vi "User Update.vi"(8 "error in (no error)":errorcluster, 10 "User Record":T2, 11 "Connection Refnum":T1) -> (0 "error out":errorcluster, 3 "dup Connection Refnum":T1)   [LabVIEW 2011]
uses:
  User Record.ctl
  SI.LIB/ODBC/SQL Controls/Connection Refnum.ctl
panel:
  out "resulting string":string
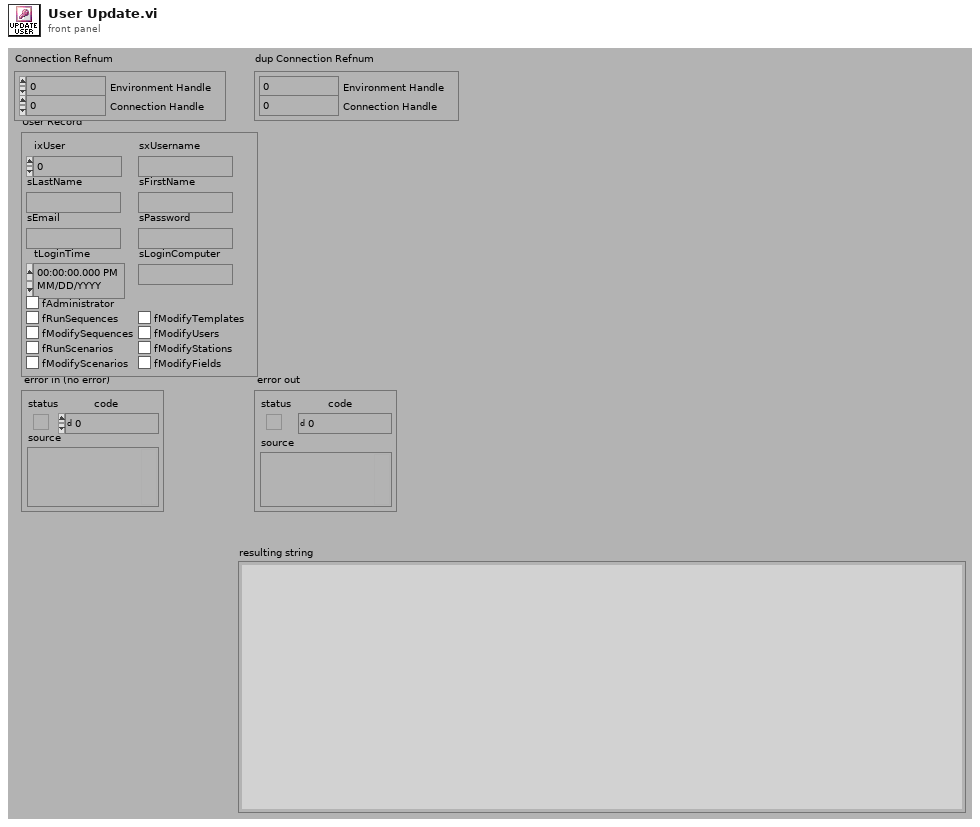
[diagram p1: front panel]
types:
  T1 = typedef "Connection Refnum.ctl" = cluster{"Environment Handle":i32, "Connection Handle":i32}
  T2 = typedef "User Record.ctl" = cluster{"ixUser":i32, "sxUsername":string, "sLastName":string, "sFirstName":string, "sEmail":string, "sPassword":string, "tLoginTime":timestamp, "sLoginComputer":string, "fAdministrator":bool, "fRunSequences":bool, "fModifySequences":bool, "fRunScenarios":bool, "fModifyScenarios":bool, "fModifyTemplates":bool, "fModifyUsers":bool, "fModifyStations":bool, "fModifyFields":bool}
  T3 = typedef "Statement Refnum.ctl" = cluster{"Statement Handle":i32, "Parameter Number":u16}
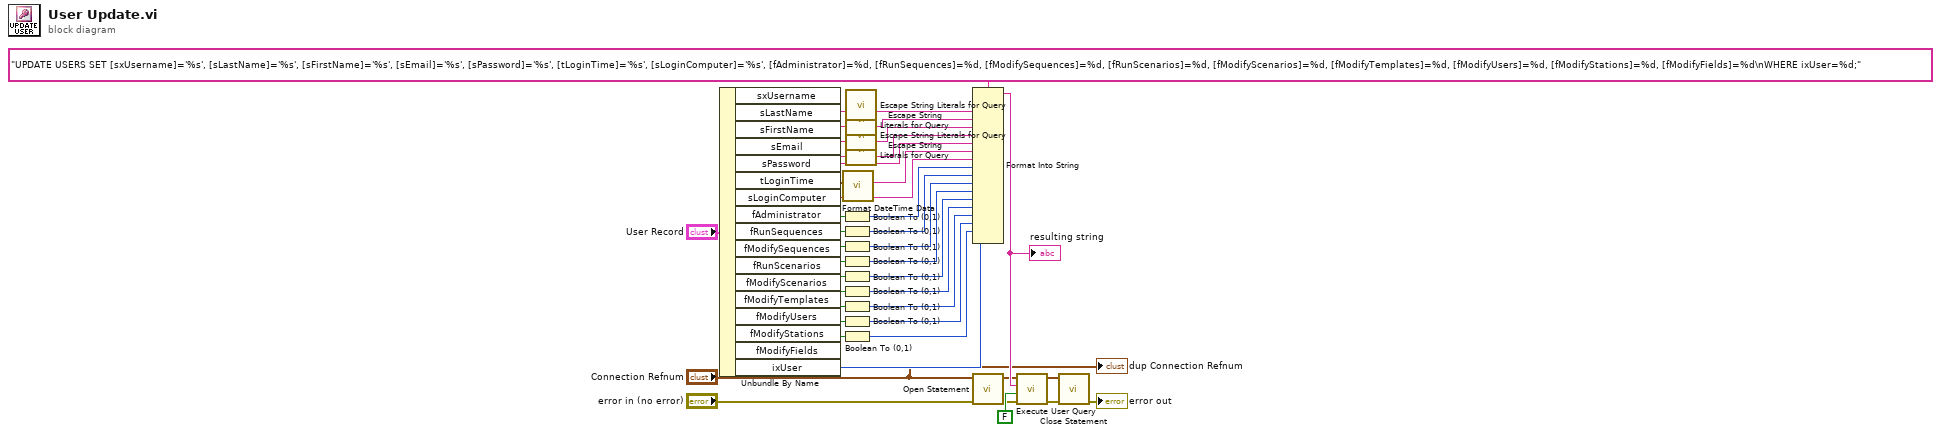
[diagram p0: block diagram]
diagram:
  n1 = Unbundle By Name("User Record") -> ("sxUsername"=w32:string, "sLastName"=w28:string, "sFirstName"=w29:string, "sEmail"=w30:string, "sPassword"=w23:string, "tLoginTime"=w27:timestamp, "sLoginComputer"=w34:string, "fAdministrator"=w20:bool, "fRunSequences"=w19:bool, "fModifySequences"=w18:bool, "fRunScenarios"=w14:bool, "fModifyScenarios"=w13:bool, "fModifyTemplates"=w12:bool, "fModifyUsers"=w11:bool, "fModifyStations"=w10:bool, "fModifyFields"=w9:bool, "ixUser"=w21:i32)
  n2 = Boolean To (0,1)(Boolean=w20) -> (0, 1=w15:i16)
  n3 = Boolean To (0,1)(Boolean=w19) -> (0, 1=w16:i16)
  n4 = Boolean To (0,1)(Boolean=w18) -> (0, 1=w17:i16)
  n5 = Boolean To (0,1)(Boolean=w14) -> (0, 1=w3:i16)
  n6 = Boolean To (0,1)(Boolean=w13) -> (0, 1=w4:i16)
  n7 = Boolean To (0,1)(Boolean=w12) -> (0, 1=w5:i16)
  n8 = Boolean To (0,1)(Boolean=w11) -> (0, 1=w6:i16)
  n9 = Boolean To (0,1)(Boolean=w10) -> (0, 1=w7:i16)
  n10 = Boolean To (0,1)(Boolean=w9) -> (0, 1=w8:i16)
  n11 = call "Format DateTime Data.vi"("Timestamp in"=w27) -> ("UTC DB String out"=w22:string)  [unwired: 10 out]
  n12 = call "Escape String Literals for Query.vi"("String"=w32) -> ("escaped String"=w31:string)  [unwired: 1 in, 13 out]
  n13 = call "Escape String Literals for Query.vi"("String"=w28) -> ("escaped String"=w26:string)  [unwired: 1 in, 13 out]
  n14 = call "Escape String Literals for Query.vi"("String"=w29) -> ("escaped String"=w25:string)  [unwired: 1 in, 13 out]
  n15 = call "Escape String Literals for Query.vi"("String"=w30) -> ("escaped String"=w24:string)  [unwired: 1 in, 13 out]
  n16 = Format Into String(format string="UPDATE USERS SET [sxUsername]='%s', [sLastName]='%s', [sFirstName]='%s', [sEmail]='%s', [sPassword]='%s', [tLoginTime]='%s', [sLoginComputer]='%s', [fAdministrator]=%d, [fRunSequences]=%d, [fModifySequences]=%d, [fRunScenarios]=%d, [fModifyScenarios]=%d, [fModifyTemplates]=%d, [fModifyUsers]=%d, [fModifyStations]=%d, [fModifyFields]=%d\nWHERE ixUser=%d;" ("User Query"), w31, w26, w25, w24, w23, w22, w34, w15, w16, w17, w3, w4, w5, w6, w7, w8, w21) -> (resulting string=w37:string)  [unwired: 2 in, 1 out]
  "resulting string" <- w37
  n17 = call "Open Statement.vi"("error in (no error)"="error in (no error)", "Connection Refnum"="Connection Refnum") -> ("error out"=w36:errorcluster, "Statement Refnum"=w35:T3)  [unwired: 4 out]
  n18 = call "Execute User Query.vi"("error in (no error)"=w36, "Return Data? (f)"=FALSE, "User Query"=w37, "Statement Refnum"=w35) -> ("error out"=w40:errorcluster, "Statement Refnum"=w39:T3)  [unwired: 2 out]
  n19 = call "Close Statement.vi"("error in (no error)"=w40, "Statement Refnum"=w39) -> ("error out"=→"error out":errorcluster)  [unwired: 5 out]
  "dup Connection Refnum" <- "Connection Refnum"
